vi "TEST optimize swerve.vi"() -> ()   [LabVIEW 2023]
uses:
  <vilib>/Analysis/coordinate.llb/Angle Range (Degree).ctl
  <vilib>/Analysis/coordinate.llb/Angle Units.ctl
  <vilib>/Analysis/coordinate.llb/Wrap Angle (scalar).vi
  <vilib>/Analysis/NI_AAL_Angle.lvlib
panel:
  out "output":T1(array[cluster])=[{"velocity out"=1.0, "POS out"=90.0, "ABS out"=90.0, "deg CCW"=90.0, "reset"=FALSE}, {"velocity out"=1.0, "POS out"=-90.0, "ABS out"=270.0, "deg CCW"=-90.0, "reset"=FALSE}, {"velocity out"=1.0, "POS out"=-10.0, "ABS out"=350.0, "deg CCW"=-20.0, "reset"=FALSE}, {"velocity out"=-1.0, "POS out"=10.0, "ABS out"=10.0, "deg CCW"=0.0, "reset"=FALSE}, {"velocity out"=1.0, "POS out"=100.0, "ABS out"=100.0, "deg CCW"=90.0, "reset"=FALSE}, {"velocity out"=0.0, "POS out"=90.0, "ABS out"=90.0, "deg CCW"=80.0, "reset"=TRUE}, {"velocity out"=-1.0, "POS out"=-50.0, "ABS out"=310.0, "deg CCW"=-5.0, "reset"=FALSE}, {"velocity out"=0.0, "POS out"=90.0, "ABS out"=90.0, "deg CCW"=85.0, "reset"=TRUE}, {"velocity out"=-1.0, "POS out"=5.0, "ABS out"=5.0, "deg CCW"=5.0, "reset"=FALSE}]
  out "delta = target - POS":dbl[](array[numeric])=[90.0, 270.0, 340.0, 180.0, 90.0, 90.0, -185.0, -5.0, 185.0]
  out "POS":dbl[](array[numeric])=[0.0, 0.0, 10.0, 10.0, 10.0, 10.0, -45.0, 5.0, 0.0]
  in  "input":T2(array[cluster])=[{"POS"=0.0, "target angle"=90.0, "velocity"=1.0}, {"POS"=0.0, "target angle"=270.0, "velocity"=1.0}, {"POS"=10.0, "target angle"=350.0, "velocity"=1.0}, {"POS"=10.0, "target angle"=190.0, "velocity"=1.0}, {"POS"=10.0, "target angle"=100.0, "velocity"=1.0}, {"POS"=10.0, "target angle"=100.0, "velocity"=0.0}, {"POS"=-45.0, "target angle"=130.0, "velocity"=1.0}, {"POS"=5.0, "target angle"=0.0, "velocity"=0.0}, {"POS"=0.0, "target angle"=185.0, "velocity"=1.0}] {"velocity" format="%_4f"; "target angle" format="%_4f"; "POS" format="%_4f"}
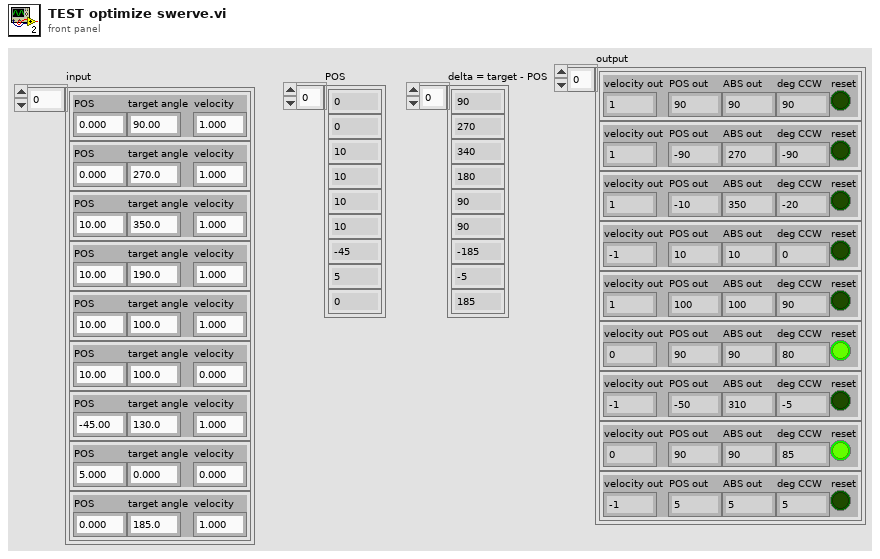
[diagram p1: front panel]
types:
  T1 = cluster{"velocity out":dbl, "POS out":dbl, "ABS out":dbl, "deg CCW":dbl, "reset":bool}[]
  T2 = cluster{"POS":dbl, "target angle":dbl, "velocity":dbl}[]
  T3 = cluster{"velocity out":dbl, "POS out":dbl, "ABS out":dbl, "deg CCW":dbl, "reset":bool}
  T4 = typedef "NI_AAL_Angle.lvlib/Angle Units.ctl" = i32
  T5 = typedef "NI_AAL_Angle.lvlib/Angle Range (Degree).ctl" = u16
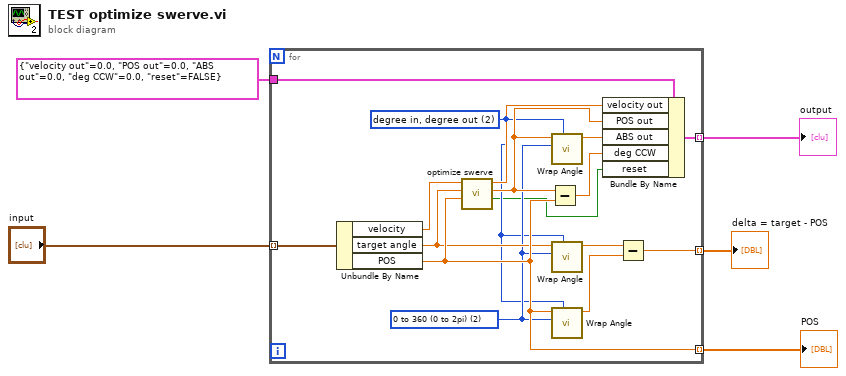
[diagram p0: block diagram]
diagram:
  n1 = for {
    tunnel: "input" -> [w21] mode=indexing
    tunnel: [w18] -> w1 mode=indexing
    tunnel: [w13] -> w4 mode=indexing
    tunnel: [w17] -> w3 mode=indexing
    tunnel: T3 {"velocity out"=0.0, "POS out"=0.0, "ABS out"=0.0, "deg CCW"=0.0, "reset"=FALSE} -> [w9]
    w7 = T4 2 items=["radian in, radian out", "radian in, degree out", "degree in, degree out", "degree in, radian out"] ("angle units")
    w8 = T5 2 items=["none", "-180 to 180 (-pi to pi)", "0 to 360 (0 to 2pi)"] ("angle range")
    n2 = Unbundle By Name(w21) -> ("velocity"=w20:dbl, "target angle"=w10:dbl, "POS"=w13:dbl)
    n3 = call "optimize swerve.vi"("current angle (deg)"=w13, "target angle (deg)"=w10, "velocity"=w20) -> ("reset POS to ABS"=w6:bool, "steer angle (deg)"=w12:dbl, "velocity"=w19:dbl)  [unwired: 5 in, 1 out]
    n4 = Subtract(x=w12, y=w13) -> (x-y=w14:dbl)
    n5 = call-poly <vilib>:"Wrap Angle.vi"("angle units"=w7, "angle range"=w8, "angle in"=w12) -> ("angle out"=w11:dbl)  [unwired: 7 in, 1 out]
    n6 = call-poly <vilib>:"Wrap Angle.vi"("angle units"=w7, "angle range"=w8, "angle in"=w10) -> ("angle out"=w16:dbl)  [unwired: 7 in, 1 out]
    n7 = call-poly <vilib>:"Wrap Angle.vi"("angle units"=w7, "angle range"=w8, "angle in"=w13) -> ("angle out"=w15:dbl)  [unwired: 7 in, 1 out]
    n8 = Bundle By Name(cluster=w9, "velocity out"=w19, "POS out"=w12, "ABS out"=w11, "deg CCW"=w14, "reset"=w6) -> (w18:T3)
    n9 = Subtract(x=w16, y=w15) -> (x-y=w17:dbl)
  }
  "POS" <- w4
  "delta = target - POS" <- w3
  "output" <- w1
